vi "notificationsLow.vi"(8 "error in (no error)":errorcluster, 11 "reference in":refnum<class "Project Panels.lvclass">=refnum) -> (0 "error out":errorcluster, 2 "saved?":bool, 3 "reference out":refnum<class "Project Panels.lvclass">)   [LabVIEW 2016, in "Project Panels.lvclass"]
uses:
  Project Panels.lvclass
  stateItem.ctl
  SYS/Devices Controller_llb/deviceType.ctl
  SYS/Devices Controller_llb/Devices Controller.lvclass
  SYS/Notification Controller_class/Notification Controller.lvclass
panel:
  out "title":string="Cosmed Asia Pacific - Notifications"
  out "notification":string[][](table)
  in  "Edit Item":bool
  in  "Send Follow Up":bool
  out "Item Selected (S/N or P/N):":string
  out "statuBar":string="Select an item and press the follow up button...."
  in  "Stop Button":bool
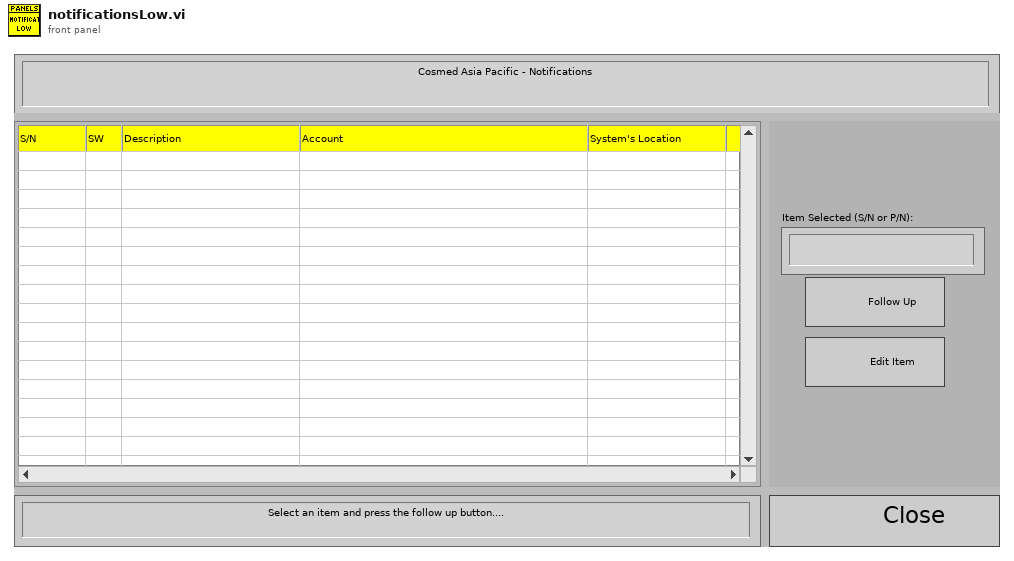
[diagram p1: front panel]
types:
  T1 = typedef "Project Panels.lvclass/stateItem.ctl" = enum16{"initiate", "waitEvent", "save", "search", "UploadFile", "nextItems", "stop"}
  T2 = typedef "Devices Controller.lvclass/deviceType.ctl" = enum16{"k5", "k4b2", "fitmate", "cpet", "rmr", "bodyBoxPft", "bp", "pp"}
  T3 = typedef "Project Panels.lvclass/ObjectAttributesRef.ctl" = refnum<data-value>
  T4 = typedef "Project Panels.lvclass/ObjectAttributes.ctl" = cluster{"MyAttribute":dbl, "device_controller_ref":refnum<class "Devices Controller.lvclass">, "file_controller_ref":refnum<class "File Controller.lvclass">, "item_controller_ref":refnum<class "Items Controller.lvclass">, "item_tables":cluster{"checkIN":string[][], "checkOUT":string[][], "storage":string[][]}, "quickbook_table":cluster{"notes":string[][]}, "notification_controller_ref":refnum<class "Notification Controller.lvclass">, "partstracking_controller_ref":refnum<class "PartsTracking Controller.lvclass">, "product_tables":cluster{"k4b2":string[][], "fitmate":string[][], "RMR":string[][], "CPET":string[][], "BP":string[][], "PP":string[][], "k5":string[][], "bb-pft":string[][]}, "rowsColour":u32[], "low_resolution?":bool, "run_python?":bool}
  T5 = enum8{"Enabled", "Disabled", "Disabled and Grayed Out"}
  T6 = typedef "LVRowAndColumnTypeDef.ctl" = cluster{"Row":i32, "Column":i32}
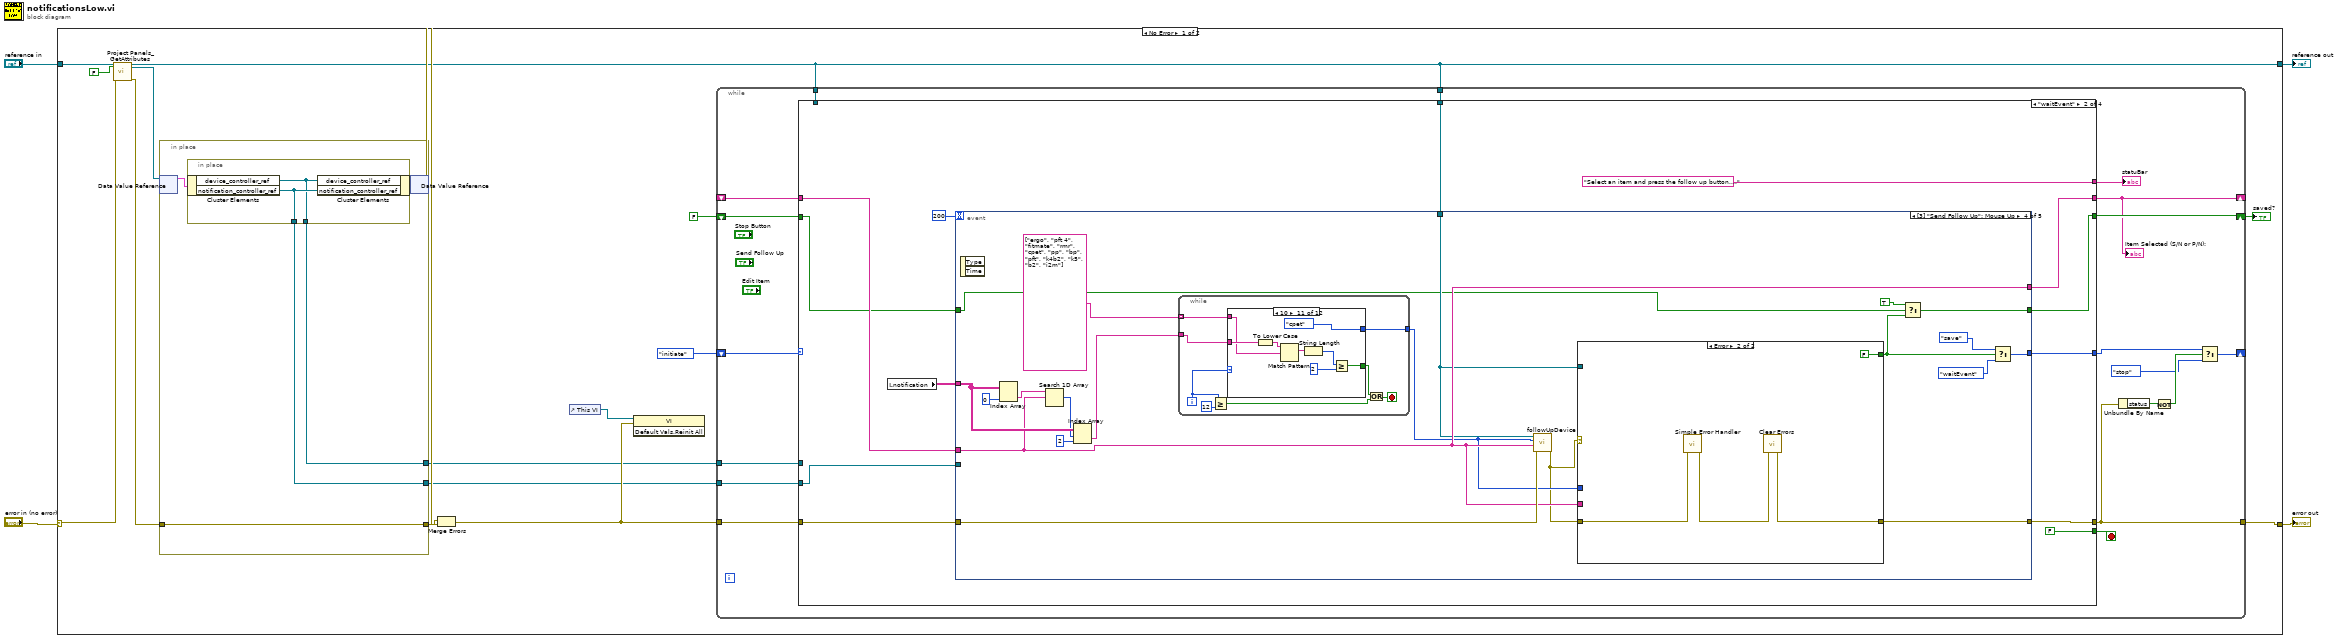
[diagram p0: block diagram]
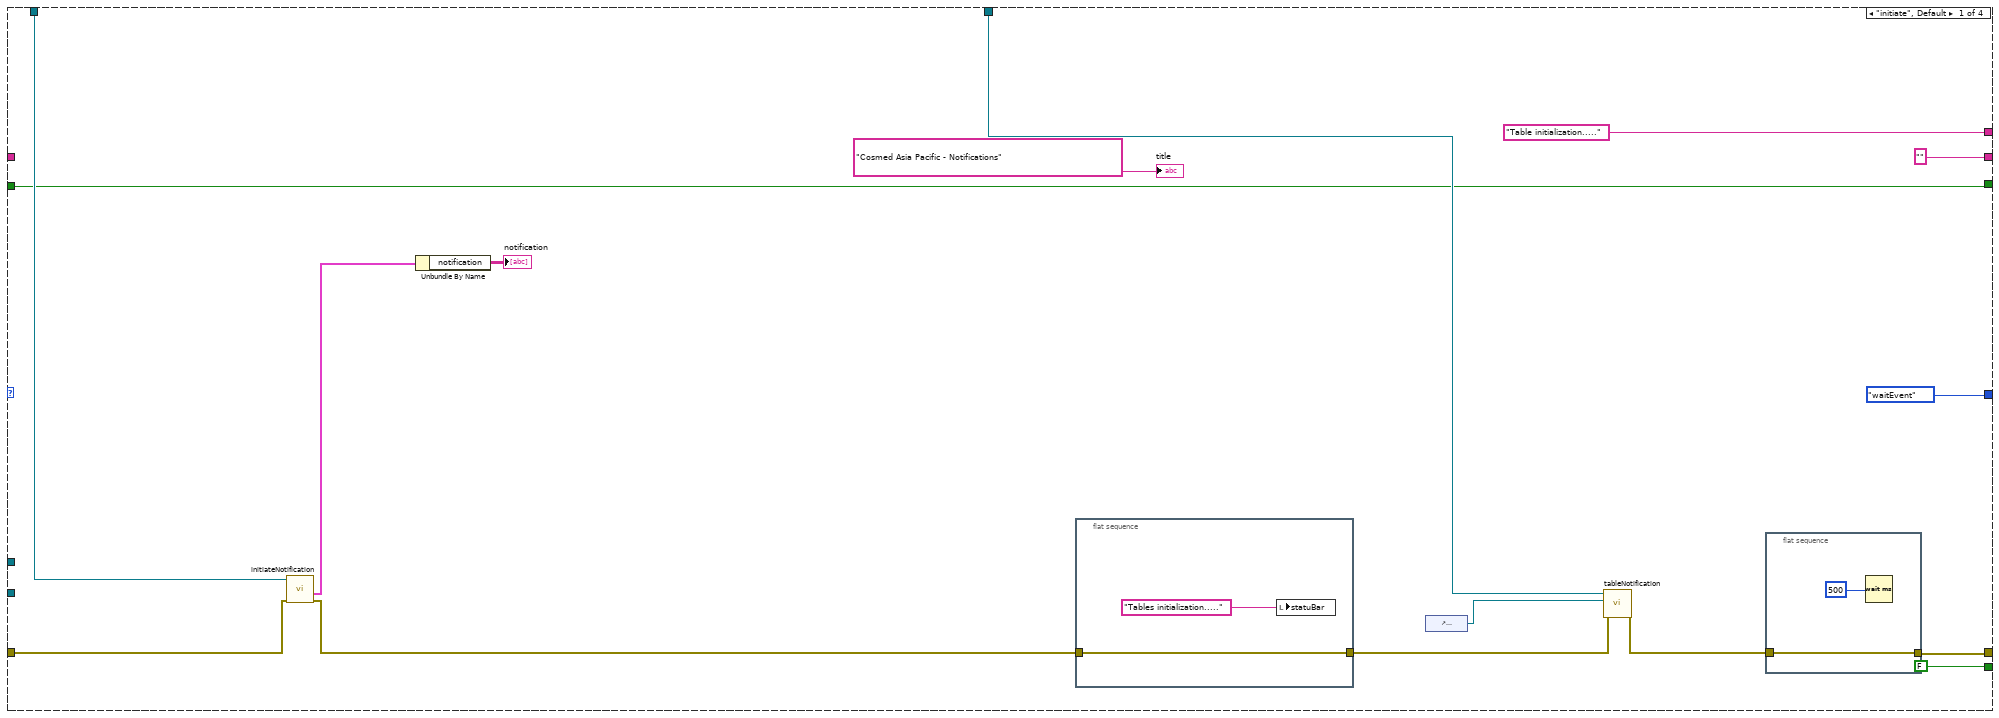
[diagram p2: hidden frame]
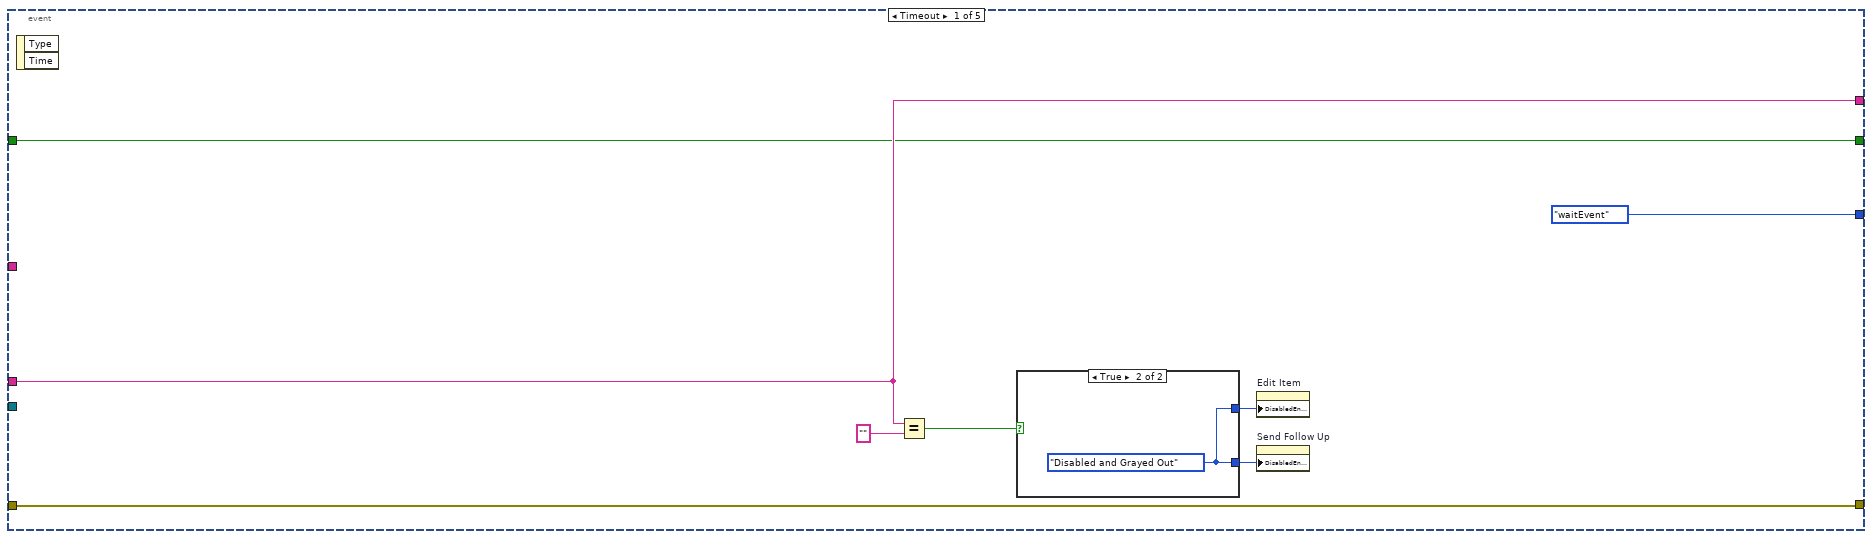
[diagram p3: hidden frame]
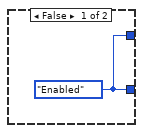
[diagram p4: hidden frame]
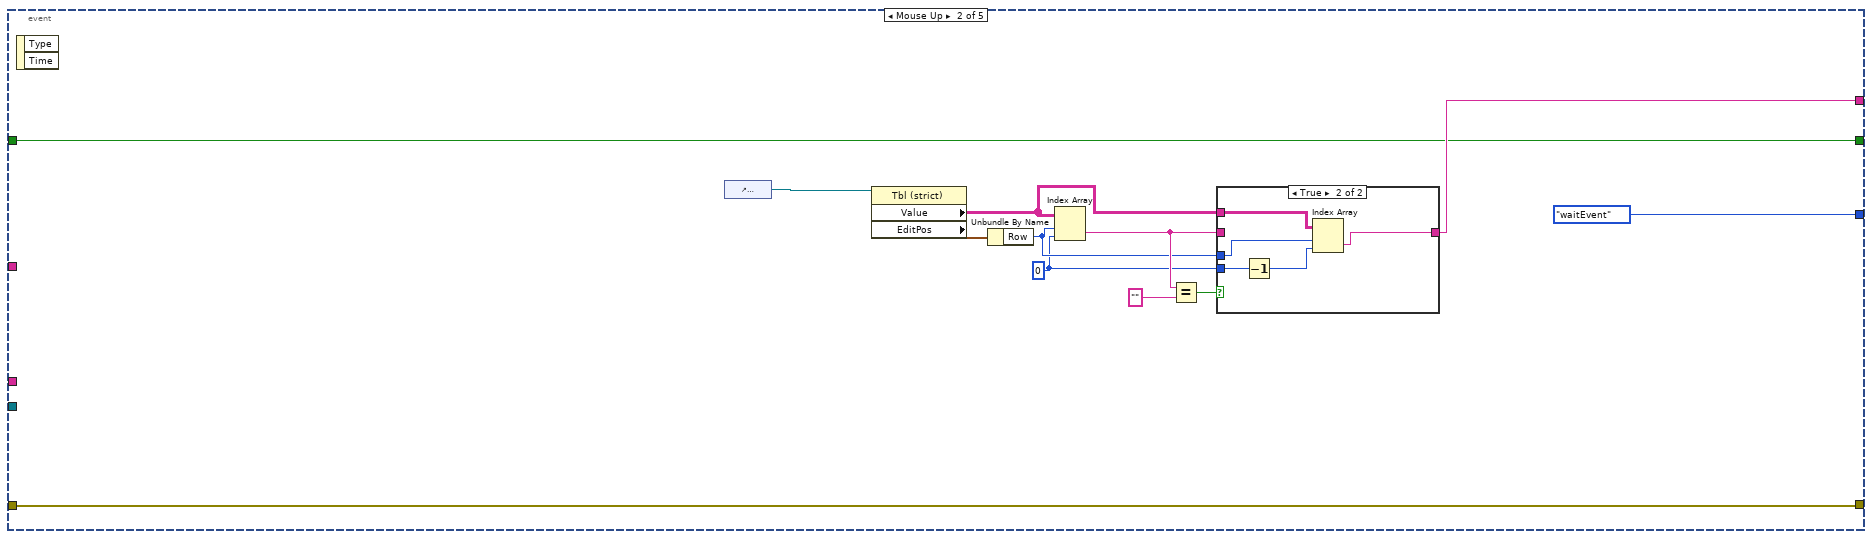
[diagram p5: hidden frame]
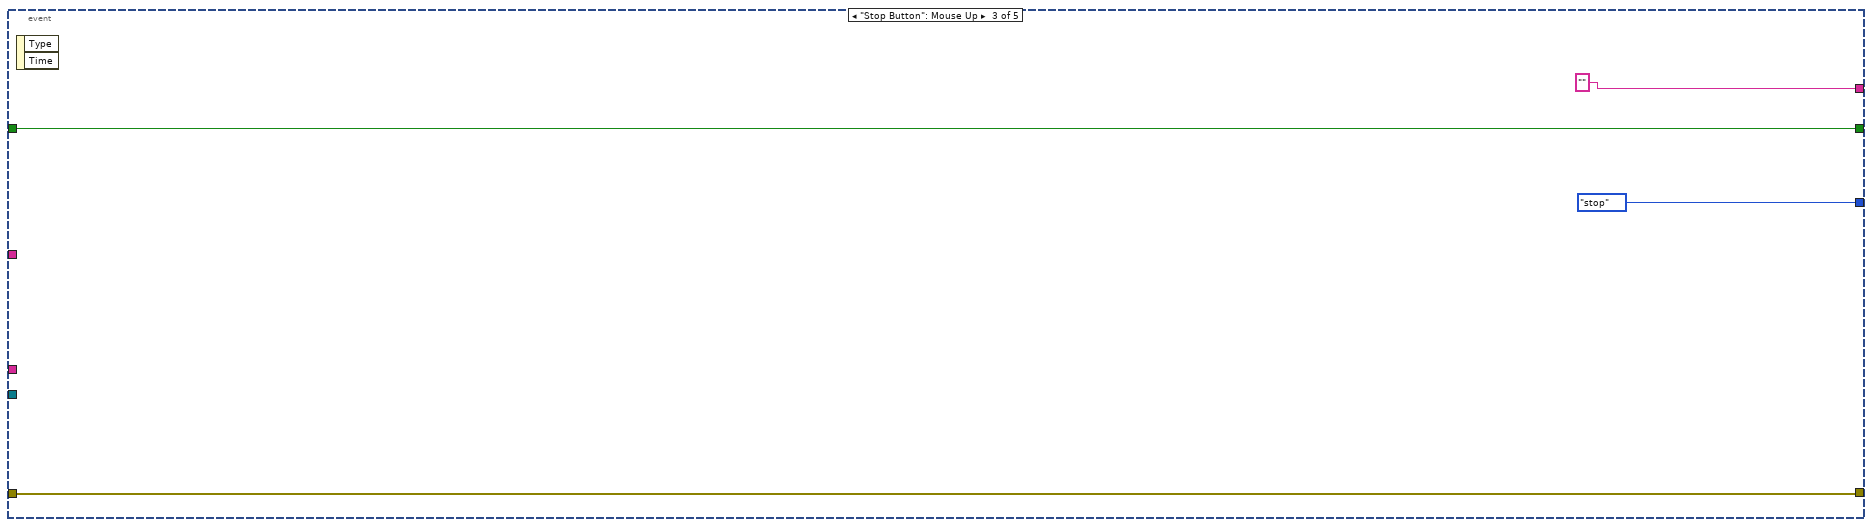
[diagram p7: hidden frame]
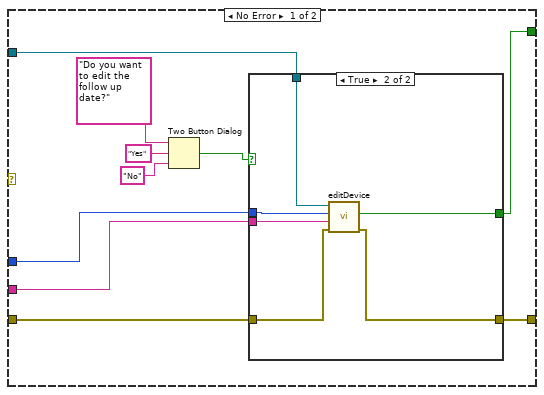
[diagram p8: hidden frame]
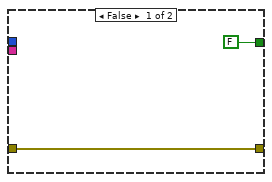
[diagram p9: hidden frame]
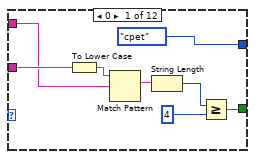
[diagram p10: hidden frame]
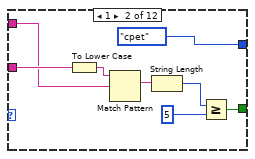
[diagram p11: hidden frame]
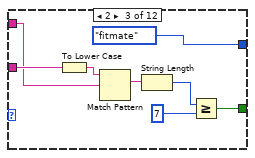
[diagram p12: hidden frame]
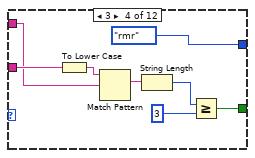
[diagram p13: hidden frame]
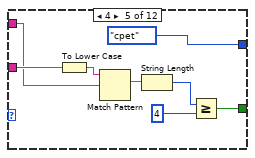
[diagram p14: hidden frame]
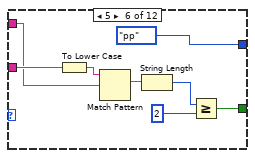
[diagram p15: hidden frame]
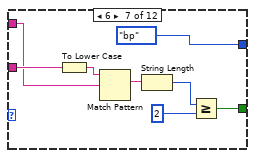
[diagram p16: hidden frame]
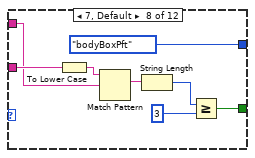
[diagram p17: hidden frame]
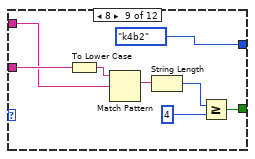
[diagram p18: hidden frame]
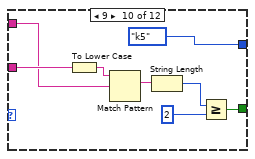
[diagram p19: hidden frame]
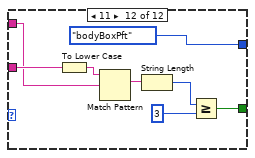
[diagram p20: hidden frame]
diagram:
  n1 = case shown="No Error" "error in (no error)" {
    selector: "error in (no error)" -> [w16 w349]
    tunnel: [w13 w349] -> w3
    tunnel: [w11 w348] -> w1
    tunnel: "reference in" -> [w18 w348]
    frame No Error {
      n2 = call "Project Panels_GetAttributes.vi"("reference in"=w18, "return data? (T)"=FALSE, "error in (no error)"=w16) -> ("reference out"=w11:refnum<class "Project Panels.lvclass">, "attributes ref"=w14:T3, "error out"=w15:errorcluster)  [unwired: 13 in, 1 out]
      n3 = in-place {
        in-place-border: w15 -> [w343]
        in-place-border: [w343] -> w19
        in-place-border: [w342] -> w8
        in-place-border: [w341] -> w5
        n4 = in-place-dvr #1(w14) -> (w344:T4)  [unwired: 1 out]
        n5 = in-place {
          in-place-border: [w347] -> w342
          in-place-border: [w346] -> w341
          n6 = in-place-cluster #2(w344) -> ("device_controller_ref"=w346:refnum<class "Devices Controller.lvclass">, "notification_controller_ref"=w347:refnum<class "Notification Controller.lvclass">)
          n7 = in-place-cluster #2("device_controller_ref"=w346, "notification_controller_ref"=w347) -> (w345:T4)
        }
        n8 = in-place-dvr #1(w345) -> (w20:errorcluster)  [unwired: 1 out]
      }
      n9 = Merge Errors(w19, w20) -> (w9:errorcluster)
      n10 = control-ref of="This VI"() -> (w10:refnum<vi>)
      n11 = invoke class="VI" method="Default Vals.Reinit All"(reference=w10, error in=w9) -> ()  [unwired: 1 in, 3 out]
      n12 = while {
        tunnel: w11 -> [w38]
        tunnel: w9 -> [w37]
        tunnel: [w35] -> w13
        shift-right: [w32] -> _
        shift-left: stateItem."initiate" ("state") -> [w36]
        shift-right: [w22] -> _
        shift-left: _ -> [w28]
        tunnel: w11 -> [w27]
        tunnel: w8 -> [w25]
        shift-right: [w23] -> w6
        shift-left: FALSE -> [w24]
        tunnel: w5 -> [w21]
        stop <- w30 stop-if-true
        n13 = case shown="\"waitEvent\"" w36 {
          tunnel: w38 -> [w48 w62 _ _]
          tunnel: w37 -> [w43 w70 w309 w319]
          tunnel: [w51 w65 w310 w318] -> w35
          tunnel: [stateItem."waitEvent" ("state") w64 stateItem."initiate" ("state") stateItem."stop" ("state")] -> w33
          tunnel: [FALSE FALSE FALSE TRUE] -> w30
          tunnel: ["Table initialization....." ("title") "Select an item and press the follow up button...." ("title") "wait" ("title") w326] -> w29
          tunnel: ["" w66 w311 w329] -> w22
          tunnel: w28 -> [_ w67 w311 w329]
          tunnel: w27 -> [w47 _ _ _]
          tunnel: w25 -> [_ w63 w312 _]
          tunnel: w24 -> [w40 w60 w308 w321]
          tunnel: [w40 w61 w308 w321] -> w23
          tunnel: w21 -> [_ _ _ w320]
          frame "initiate", Default {
            n14 = call "initiateNotification.vi"("error in (no error)"=w43, "reference in"=w47) -> ("error out"=w45:errorcluster, "table"=w46:cluster{"notification":string[][]})  [unwired: 7 in, 1 out]
            n15 = Unbundle By Name(w46) -> ("notification"=→"notification":string[][])
            n16 = flat-sequence {
              tunnel: w45 -> [w56]
              tunnel: [w56] -> w50
              frame #0 {
                n17 = local write "statuBar"("Tables initialization....." ("title")) -> ()
              }
            }
            n18 = control-ref of="notification"() -> (w41:refnum<vi>)
            n19 = call "tableNotification.vi"("error in (no error)"=w50, "Table in"=w41, "reference in"=w48) -> ("error out"=w42:errorcluster)  [unwired: 7 in, 1 out]
            n20 = flat-sequence {
              tunnel: w42 -> [w58]
              tunnel: [w58] -> w51
              frame #0 {
                n21 = Wait (ms)(milliseconds to wait=u32 500) -> ()  [unwired: 1 out]
              }
            }
            "title" <- "Cosmed Asia Pacific - Notifications" ("title")
          }
          frame "waitEvent" {
            n22 = local read "notification"() -> (w59:string[][])
            n23 = event shown="[3] \"Send Follow Up\": Mouse Up" {
              selector: _ -> [_ _ _ _ _]
              dyn-events: _ -> [_ _ _ _ _]
              timeout: 200 -> [_ _ _ _ _]
              tunnel: w70 -> [w79 w93 w103 w123 w268]
              tunnel: [w79 w93 w103 w116 w252] -> w65
              tunnel: w67 -> [w76 _ _ w115 w263]
              tunnel: [w76 w84 "" w115 w263] -> w66
              tunnel: [stateItem."waitEvent" ("state") stateItem."waitEvent" ("state") stateItem."stop" ("state") w110 w258] -> w64
              tunnel: w63 -> [_ _ _ _ w251]
              tunnel: w62 -> [_ _ _ w113 w269]
              tunnel: w59 -> [_ _ _ w120 w262]
              tunnel: [w72 w82 w100 w107 w255] -> w61
              tunnel: w60 -> [w72 w82 w100 w106 w254]
              event Timeout {
                n24 = event-data() -> ()  [unwired: 1 in, 2 out]
                n25 = Equal?(x=w76, y="") -> (x = y?=w78:bool)
                n26 = case shown="True" w78 {
                  tunnel: [w80 w81] -> w74
                  tunnel: [w80 w81] -> w73
                  frame False {
                    w80 = T5."Enabled" ("Disabled")
                  }
                  frame True {
                    w81 = T5."Disabled and Grayed Out" ("Disabled")
                  }
                }
                n27 = property on="Edit Item" class="Bool"("DisabledEnum"=w73) -> ()  [unwired: 2 in, 2 out]
                n28 = property on="Send Follow Up" class="Bool (strict)"("DisabledEnum"=w74) -> ()  [unwired: 2 in, 2 out]
              }
              event Mouse Up {
                w85 = 0 ("disabled index (col)")
                n29 = event-data() -> ()  [unwired: 1 in, 2 out]
                n30 = control-ref of="notification"() -> (w91:refnum<vi>)
                n31 = property on="Property Node" class="Tbl (strict)"(reference=w91) -> ("Value"=w87:string[][], "EditPos"=w92:T6)  [unwired: 1 in, 2 out]
                n32 = Unbundle By Name(w92) -> ("Row"=w86:i32)
                n33 = Index Array(array=w87, index (row)=w86, index (col)=w85) -> (element=w88:string)
                n34 = Equal?(x=w88, y="") -> (x = y?=w89:bool)
                n35 = case shown="True" w89 {
                  tunnel: w88 -> [w94 _]
                  tunnel: [w94 w95] -> w84
                  tunnel: w87 -> [_ w99]
                  tunnel: w86 -> [_ w98]
                  tunnel: w85 -> [_ w97]
                  frame False {
                  }
                  frame True {
                    n36 = Decrement(x=w97) -> (x-1=w96:i32)
                    n37 = Index Array(array=w99, index (row)=w98, index (col)=w96) -> (element=w95:string)
                  }
                }
              }
              event "Stop Button": Mouse Up {
                n38 = event-data() -> ()  [unwired: 1 in, 2 out]
              }
              event "Send Follow Up": Mouse Up {
                n39 = event-data() -> ()  [unwired: 1 in, 2 out]
                n40 = Index Array(array=w120, index (col)=0 ("disabled index (col)")) -> (element=w121:string[])  [unwired: 1 in]
                n41 = Search 1D Array(1D array=w121, element=w115) -> (index of element=w119:i32)  [unwired: 1 in]
                n42 = Index Array(array=w120, index (row)=w119, index (col)=2 ("disabled index (col)")) -> (element=w117:string)
                n43 = while {
                  tunnel: w117 -> [w153]
                  tunnel: [w152] -> w114
                  tunnel: string[] ["ergo", "pft 4", "fitmate", "rmr", "cpet", "pp", "bp", "pft", "k4b2", "k5", "b2", "i2m"] -> [w151] mode=indexing
                  i -> [w148]
                  stop <- w149 stop-if-true
                  n44 = Greater Or Equal?(x=w148, y=12) -> (x >= y?=w146:bool)
                  n45 = case shown="10" w148 {
                    tunnel: w153 -> [w157 w165 w177 w185 w193 w201 w209 w217 w221 w229 w241 w249]
                    tunnel: [w156 w164 w176 w184 w192 w200 w208 w216 w220 w228 w240 w248] -> w150
                    tunnel: [deviceType."cpet" ("deviceType") deviceType."cpet" ("deviceType") deviceType."fitmate" ("deviceType") deviceType."rmr" ("deviceType") deviceType."cpet" ("deviceType") deviceType."pp" ("deviceType") deviceType."bp" ("deviceType") deviceType."bodyBoxPft" ("deviceType") deviceType."k4b2" ("deviceType") deviceType."k5" ("deviceType") deviceType."cpet" ("deviceType") deviceType."bodyBoxPft" ("deviceType")] -> w152
                    tunnel: w151 -> [w154 w162 w170 w178 w186 w194 w202 w210 w218 w226 w234 w242]
                    frame 0 {
                      n46 = To Lower Case(string=w157) -> (all lower case string=w158:string)
                      n47 = Match Pattern(string=w158, regular expression=w154) -> (match substring=w159:string)  [unwired: 1 in, 3 out]
                      n48 = String Length(string=w159) -> (length=w160:i32)
                      n49 = Greater Or Equal?(x=w160, y=4) -> (x >= y?=w156:bool)
                    }
                    frame 1 {
                      n50 = To Lower Case(string=w165) -> (all lower case string=w166:string)
                      n51 = Match Pattern(string=w166, regular expression=w162) -> (match substring=w167:string)  [unwired: 1 in, 3 out]
                      n52 = String Length(string=w167) -> (length=w168:i32)
                      n53 = Greater Or Equal?(x=w168, y=5) -> (x >= y?=w164:bool)
                    }
                    frame 2 {
                      n54 = To Lower Case(string=w177) -> (all lower case string=w171:string)
                      n55 = Match Pattern(string=w171, regular expression=w170) -> (match substring=w172:string)  [unwired: 1 in, 3 out]
                      n56 = String Length(string=w172) -> (length=w173:i32)
                      n57 = Greater Or Equal?(x=w173, y=7) -> (x >= y?=w176:bool)
                    }
                    frame 3 {
                      n58 = To Lower Case(string=w185) -> (all lower case string=w179:string)
                      n59 = Match Pattern(string=w179, regular expression=w178) -> (match substring=w180:string)  [unwired: 1 in, 3 out]
                      n60 = String Length(string=w180) -> (length=w181:i32)
                      n61 = Greater Or Equal?(x=w181, y=3) -> (x >= y?=w184:bool)
                    }
                    frame 4 {
                      n62 = To Lower Case(string=w193) -> (all lower case string=w187:string)
                      n63 = Match Pattern(string=w187, regular expression=w186) -> (match substring=w188:string)  [unwired: 1 in, 3 out]
                      n64 = String Length(string=w188) -> (length=w189:i32)
                      n65 = Greater Or Equal?(x=w189, y=4) -> (x >= y?=w192:bool)
                    }
                    frame 5 {
                      n66 = To Lower Case(string=w201) -> (all lower case string=w195:string)
                      n67 = Match Pattern(string=w195, regular expression=w194) -> (match substring=w196:string)  [unwired: 1 in, 3 out]
                      n68 = String Length(string=w196) -> (length=w197:i32)
                      n69 = Greater Or Equal?(x=w197, y=2) -> (x >= y?=w200:bool)
                    }
                    frame 6 {
                      n70 = To Lower Case(string=w209) -> (all lower case string=w203:string)
                      n71 = Match Pattern(string=w203, regular expression=w202) -> (match substring=w204:string)  [unwired: 1 in, 3 out]
                      n72 = String Length(string=w204) -> (length=w205:i32)
                      n73 = Greater Or Equal?(x=w205, y=2) -> (x >= y?=w208:bool)
                    }
                    frame 7, Default {
                      n74 = To Lower Case(string=w217) -> (all lower case string=w211:string)
                      n75 = Match Pattern(string=w211, regular expression=w210) -> (match substring=w212:string)  [unwired: 1 in, 3 out]
                      n76 = String Length(string=w212) -> (length=w213:i32)
                      n77 = Greater Or Equal?(x=w213, y=3) -> (x >= y?=w216:bool)
                    }
                    frame 8 {
                      n78 = To Lower Case(string=w221) -> (all lower case string=w222:string)
                      n79 = Match Pattern(string=w222, regular expression=w218) -> (match substring=w223:string)  [unwired: 1 in, 3 out]
                      n80 = String Length(string=w223) -> (length=w224:i32)
                      n81 = Greater Or Equal?(x=w224, y=4) -> (x >= y?=w220:bool)
                    }
                    frame 9 {
                      n82 = To Lower Case(string=w229) -> (all lower case string=w230:string)
                      n83 = Match Pattern(string=w230, regular expression=w226) -> (match substring=w231:string)  [unwired: 1 in, 3 out]
                      n84 = String Length(string=w231) -> (length=w232:i32)
                      n85 = Greater Or Equal?(x=w232, y=2) -> (x >= y?=w228:bool)
                    }
                    frame 10 {
                      n86 = To Lower Case(string=w241) -> (all lower case string=w235:string)
                      n87 = Match Pattern(string=w235, regular expression=w234) -> (match substring=w236:string)  [unwired: 1 in, 3 out]
                      n88 = String Length(string=w236) -> (length=w237:i32)
                      n89 = Greater Or Equal?(x=w237, y=2) -> (x >= y?=w240:bool)
                    }
                    frame 11 {
                      n90 = To Lower Case(string=w249) -> (all lower case string=w243:string)
                      n91 = Match Pattern(string=w243, regular expression=w242) -> (match substring=w244:string)  [unwired: 1 in, 3 out]
                      n92 = String Length(string=w244) -> (length=w245:i32)
                      n93 = Greater Or Equal?(x=w245, y=3) -> (x >= y?=w248:bool)
                    }
                  }
                  n94 = Or(x=w150, y=w146) -> (x .or. y?=w149:bool)
                }
                n95 = call "followUpDevice.vi"("error in (no error)"=w123, "S/N"=w115, "Device Type"=w114, "reference in"=w113) -> ("error out"=w105:errorcluster)  [unwired: 6 in, 1 out]
                n96 = case shown="Error" w105 {
                  tunnel: w105 -> [w130 w144]
                  tunnel: [w129 w142] -> w116
                  tunnel: w115 -> [w127 _]
                  tunnel: w114 -> [w126 _]
                  tunnel: w113 -> [w125 _]
                  tunnel: [w124 FALSE ("saved?")] -> w108
                  frame No Error {
                    n97 = Two Button Dialog(message="Do you want to edit the follow up date?", 1:"No" ("F button name (\"Cancel\")"), 2:"Yes" ("T button name (\"OK\")")) -> (T button?=w128:bool)
                    n98 = case shown="True" w128 {
                      tunnel: w130 -> [w135 w141]
                      tunnel: [w135 w140] -> w129
                      tunnel: w127 -> [_ w139]
                      tunnel: w126 -> [_ w138]
                      tunnel: w125 -> [_ w137]
                      tunnel: [FALSE ("saved?") w136] -> w124
                      frame False {
                      }
                      frame True {
                        n99 = call "editDevice.vi"("error in (no error)"=w141, "S/N IN"=w139, "Device Type In"=w138, "reference in"=w137) -> ("error out"=w140:errorcluster, "saved?"=w136:bool)  [unwired: 5 in, 1 out]
                      }
                    }
                  }
                  frame Error {
                    n100 = call <vilib>:"Simple Error Handler.vi"("error in (no error)"=w144) -> ("error out"=w143:errorcluster)  [unwired: 4 in, 4 out]
                    n101 = call <vilib>:"Clear Errors.vi"("error in (no error)"=w143) -> ("error out"=w142:errorcluster)  [unwired: 5 in, 1 out]
                  }
                }
                n102 = Select(t=TRUE ("saved?"), s=w106, f=w108) -> (s? t:f=w107:bool)
                n103 = Select(t=stateItem."save" ("state"), s=w108, f=stateItem."waitEvent" ("state")) -> (s? t:f=w110:T1)
              }
              event "Edit Item": Mouse Up {
                n104 = event-data() -> ()  [unwired: 1 in, 3 out]
                n105 = Index Array(array=w262, index (col)=0 ("disabled index (col)")) -> (element=w266:string[])  [unwired: 1 in]
                n106 = Search 1D Array(1D array=w266, element=w263) -> (index of element=w265:i32)  [unwired: 1 in]
                n107 = Index Array(array=w262, index (row)=w265, index (col)=2 ("disabled index (col)")) -> (element=w261:string)
                n108 = while {
                  tunnel: w261 -> [w276]
                  tunnel: [w274] -> w260
                  i -> [w277]
                  stop <- w275 stop-if-true
                  n109 = case shown="3" w277 {
                    tunnel: [w280 w287 w295 TRUE] -> w275
                    tunnel: w276 -> [w279 w288 w296 w303]
                    tunnel: [deviceType."cpet" ("deviceType") deviceType."rmr" ("deviceType") deviceType."bodyBoxPft" ("deviceType") w302] -> w274
                    frame 0, Default {
                      n110 = To Lower Case(string=w279) -> (all lower case string=w281:string)
                      n111 = Match Pattern(string=w281, regular expression="quark") -> (match substring=w283:string)  [unwired: 1 in, 3 out]
                      n112 = String Length(string=w283) -> (length=w284:i32)
                      n113 = Greater Or Equal?(x=w284, y=5) -> (x >= y?=w280:bool)
                    }
                    frame 1 {
                      n114 = To Lower Case(string=w288) -> (all lower case string=w293:string)
                      n115 = Match Pattern(string=w293, regular expression="rmr") -> (match substring=w291:string)  [unwired: 1 in, 3 out]
                      n116 = String Length(string=w291) -> (length=w290:i32)
                      n117 = Greater Or Equal?(x=w290, y=3) -> (x >= y?=w287:bool)
                    }
                    frame 2 {
                      n118 = To Lower Case(string=w296) -> (all lower case string=w301:string)
                      n119 = Match Pattern(string=w301, regular expression="bp") -> (match substring=w299:string)  [unwired: 1 in, 3 out]
                      n120 = String Length(string=w299) -> (length=w298:i32)
                      n121 = Greater Or Equal?(x=w298, y=2) -> (x >= y?=w295:bool)
                    }
                    frame 3 {
                      n122 = case shown="\"K4b2\"" w303 {
                        tunnel: [deviceType."fitmate" ("deviceType") deviceType."k4b2" ("deviceType") deviceType."bp" ("deviceType")] -> w302
                        frame "Fitmate", Default {
                        }
                        frame "K4b2" {
                        }
                        frame "PP" {
                        }
                      }
                    }
                  }
                }
                n123 = call "editDevice.vi"("error in (no error)"=w268, "S/N IN"=w263, "Device Type In"=w260, "reference in"=w269) -> ("error out"=w253:errorcluster, "saved?"=w250:bool)  [unwired: 5 in, 1 out]
                n124 = Select(t=TRUE ("saved?"), s=w254, f=w250) -> (s? t:f=w255:bool)
                n125 = case shown="True" w250 {
                  tunnel: w253 -> [w270 w273]
                  tunnel: [w270 w272] -> w252
                  tunnel: w251 -> [_ w271]
                  frame False {
                  }
                  frame True {
                    n126 = call "re-initiate.vi"("reference in"=w271, "error in (no error)"=w273) -> ("error out"=w272:errorcluster)  [unwired: 16 in, 1 out]
                  }
                }
                n127 = Select(t=stateItem."initiate" ("state"), s=w250, f=stateItem."waitEvent") -> (s? t:f=w258:T1)
              }
            }
          }
          frame "save" {
            n128 = flat-sequence {
              tunnel: w309 -> [_]
              frame #0 {
                n129 = local write "statuBar"("Notification updating...." ("statuBar")) -> ()
                n130 = Wait (ms)(milliseconds to wait=u32 1000) -> ()  [unwired: 1 out]
              }
            }
            n131 = call "deleteNot.vi"("error in (no error)"=w309, "S/N:"=w311, "reference in"=w312) -> ("error out"=w310:errorcluster)  [unwired: 7 in, 1 out]
          }
          frame "stop" {
            n132 = case shown="True" w321 {
              tunnel: w319 -> [w330 w333]
              tunnel: [w330 w334] -> w318
              tunnel: w320 -> [_ w331]
              frame False {
              }
              frame True {
                n133 = flat-sequence {
                  tunnel: w333 -> [w335]
                  tunnel: [w335] -> w332
                  frame #0 {
                    n134 = local write "statuBar"("Wait....I'm saving the new data on the excel file" ("statuBar")) -> ()
                  }
                }
                n135 = call "saveData.vi"("error in (no error)"=w332, "reference in"=w331) -> ("error out"=w334:errorcluster)  [unwired: 8 in, 1 out]
              }
            }
            n136 = Unbundle By Name(w318) -> ("status"=w325:bool)
            n137 = Not(x=w325) -> (.not. x?=w324:bool)
            n138 = case shown="True" w325 {
              tunnel: w318 -> [_ w338]
              frame False {
              }
              frame True {
                n139 = Unbundle By Name(w338) -> ("source"=w337:string)
                n140 = Concatenate Strings("An Error occur: " ("message"), w337) -> (w340:string)
                n141 = One Button Dialog(message=w340) -> ()  [unwired: 1 in, 1 out]
              }
            }
            n142 = Select(t="Stoped from User" ("title"), s=w324, f="Stoped for an Error" ("title")) -> (s? t:f=w326:string)
          }
        }
        "statuBar" <- w29
        "Item Selected (S/N or P/N):" <- w22
        n143 = Unbundle By Name(w35) -> ("status"=w34:bool)
        n144 = Not(x=w34) -> (.not. x?=w31:bool)
        n145 = Select(t=w33, s=w31, f=stateItem."stop" ("state")) -> (s? t:f=w32:T1)
      }
      "saved?" <- w6
    }
    frame Error {
    }
  }
  "error out" <- w3
  "reference out" <- w1
